vi "FP Server.vi"(8 "error in":errorcluster, 11 "FP Management In":refnum<class "Front Panel Manager.lvclass">) -> (0 "error out":errorcluster, 3 "FP Management Out":refnum<class "Front Panel Manager.lvclass">)   [LabVIEW 2015, in "Front Panel Publisher.lvlib" / "Front Panel Manager.lvclass"]
uses:
  Front Panel Manager.lvclass
  Websocket_class/Websocket.lvclass
  <vilib>/wsapi/NI_WebServices.lvlib
  Connection ID Methods.ctl
  FP Server Message.ctl
  Web Front Panel_class/Web Front Panel.lvclass
  <userlib>/_OpenG.lib/array/array.llb/Conditional Auto-Indexing Tunnel (String)__ogtk.vi
  <userlib>/_OpenG.lib/array/array.llb/Conditional Auto-Indexing Tunnel (U64)__ogtk.vi
panel:
  out "Stop Loop":bool
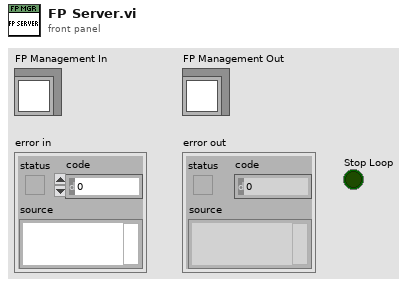
[diagram p1: front panel]
types:
  T1 = typedef "Front Panel Publisher.lvlib/Front Panel Manager.lvclass/Connection ID Methods.ctl" = enum16{"Read Data", "Write Connection ID", "Remove Connection ID"}
  T2 = typedef "Front Panel Publisher.lvlib/Front Panel Manager.lvclass/FP Server Message.ctl" = cluster{"Message":string, "Page":string, "Data":string[][], "Connection ID":u64, "Values and Position":refnum<vi>[]}
  T3 = typedef "FrontPanelPublisher.lvlib/FrontPanelManager.lvclass/FPServerMessage.ctl" = cluster{"Message":string, "Page":string, "Data":string[][], "Connection ID":u64, "Values and Position":refnum<vi>[]}
  T4 = typedef "Front Panel Publisher.lvlib/Web Front Panel.lvclass/High Level Config Settings.ctl" = cluster{"Default Refresh Rate (ms)":i32, "Show Border":bool, "Decorations Can Change":bool, "Synchronous Requests":bool, "Reduce Sent Data":bool}
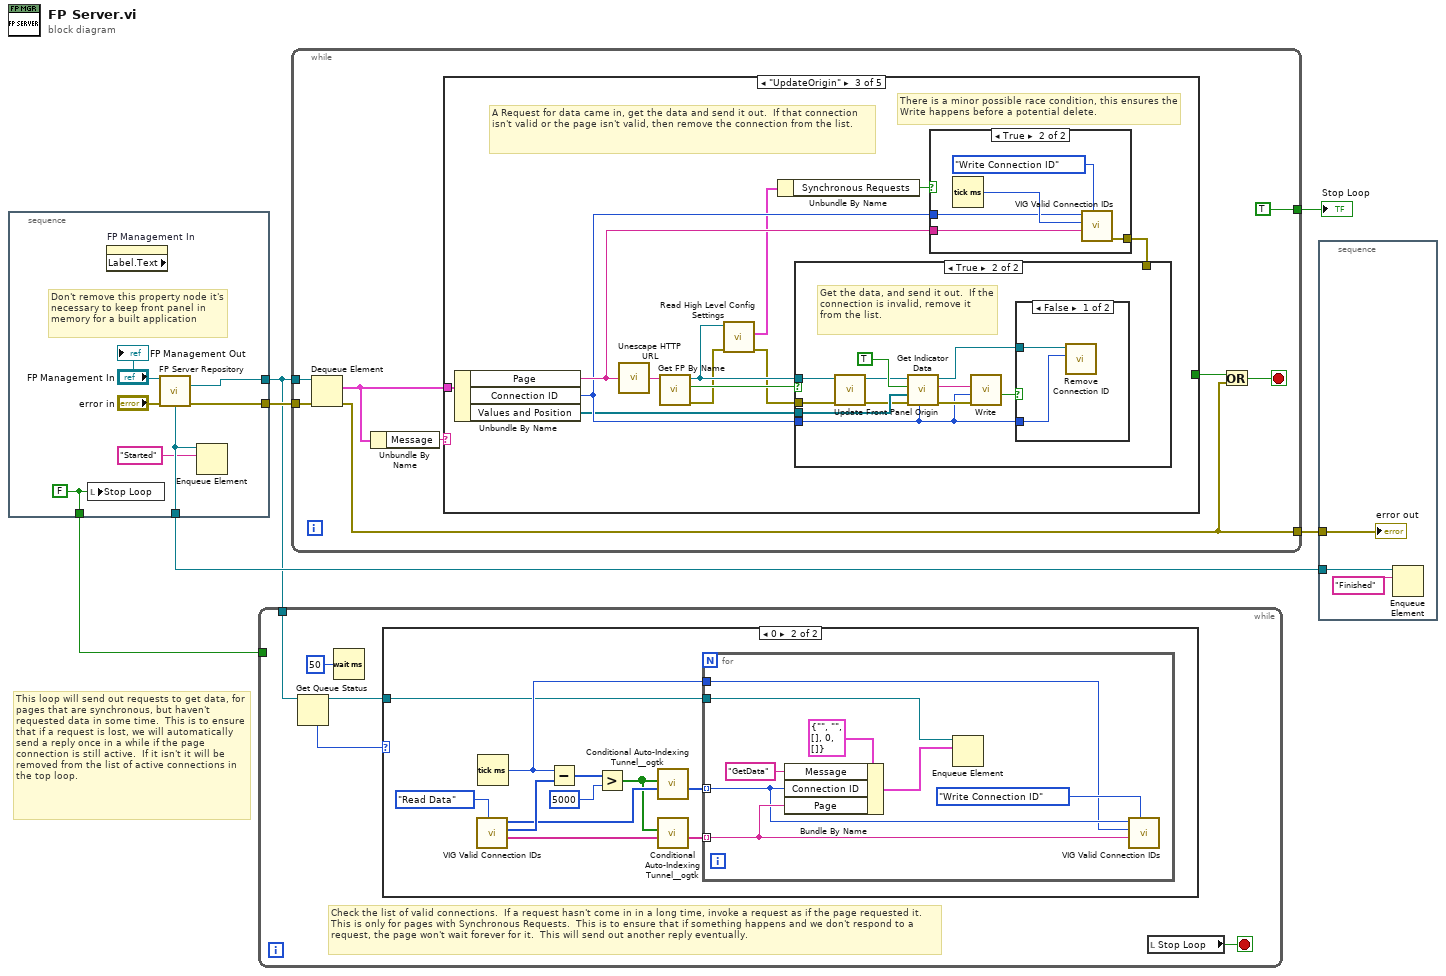
[diagram p0: block diagram]
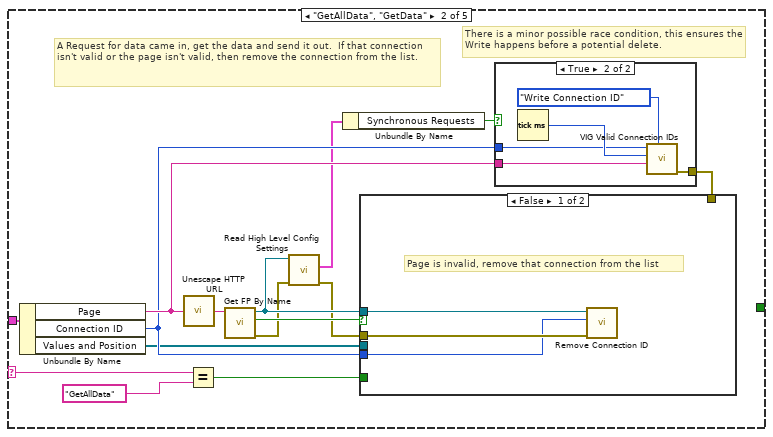
[diagram p3: hidden frame]
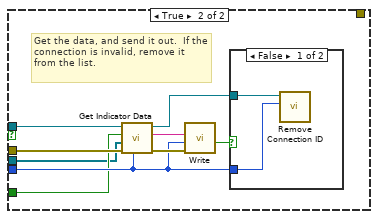
[diagram p5: hidden frame]
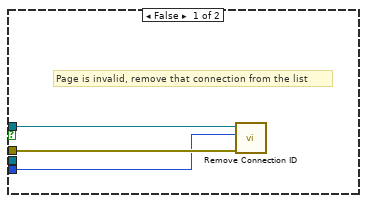
[diagram p8: hidden frame]
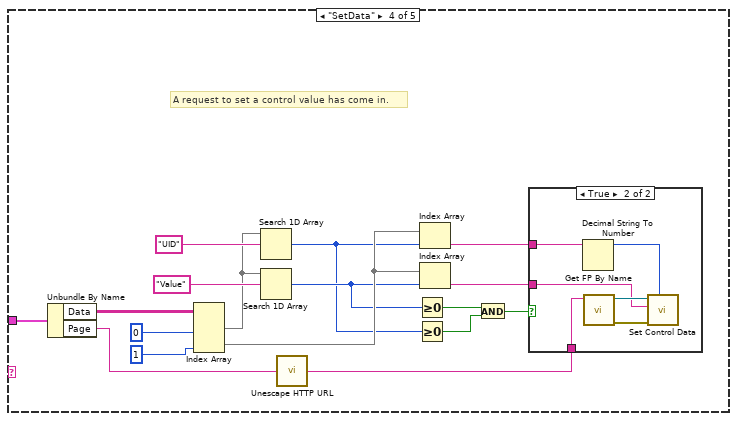
[diagram p10: hidden frame]
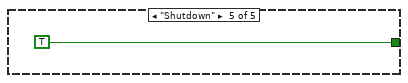
[diagram p12: hidden frame]
diagram:
  # "This loop will send out requests to get data, for pages that are synchronous, but haven't requested data in some time.  This is to ensure that if a request is lost, we will automatically send a reply once in a while if the page connection is still active.  If it isn't it will be removed from the list of active connections in the top loop."
  n1 = stacked-sequence {
    tunnel: [w11] -> w6
    tunnel: [w10] -> w3
    tunnel: [w8] -> w2
    tunnel: [w7] -> w4
    frame #0 {
      w7 = FALSE ("Stop Loop")
      # "Don't remove this property node it's necessary to keep front panel in memory for a built application"
      n2 = local write "Stop Loop"(w7) -> ()
      n3 = property on="FP Management In" class="LVClassControl (strict)" props=["Label", "Text"]() -> ()  [unwired: 2 in, 3 out]
      n4 = call "FP Server Repository.vi"("FP Management In"="FP Management In", "error in (no error)"="error in") -> ("ToProcessQueue"=w8:refnum<queue>, "ProcessSyncQueue"=w10:refnum<queue>, "error out"=w11:errorcluster)  [unwired: 7 in, 4 out]
      n5 = Enqueue Element(queue=w10, element="Started") -> ()  [unwired: 2 in, 3 out]
      "FP Management Out" <- "FP Management In"
    }
  }
  n6 = while {
    tunnel: w4 -> [_]
    tunnel: w2 -> [w16]
    stop <- w18 stop-if-true
    # "Check the list of valid connections.  If a request hasn't come in in a long time, invoke a request as if the page requested it.  This is only for pages with Synchronous Requests.  This is to ensure that if something happens and we don't respond to a request, the page won't wait forever for it.  This will send out another reply eventually."
    n7 = Get Queue Status(queue=w16) -> (queue out=w15:refnum<queue>, # elements in queue=w14:i32)  [unwired: 2 in, 6 out]
    n8 = Wait (ms)(milliseconds to wait=u32 50) -> ()  [unwired: 1 out]
    n9 = case shown="0" w14 {
      tunnel: w15 -> [_ w19]
      frame Default {
      }
      frame 0 {
        n10 = call "VIG Valid Connection IDs.vi"("Method (Read)"=Connection_ID_Methods."Read Data") -> ("Pages"=w22:string[], "Ticks"=w29:u32[], "Connections"=w26:u64[])  [unwired: 7 in, 1 out]
        n11 = Tick Count (ms)() -> (millisecond timer value=w20:u32)
        n12 = Subtract(x=w20, y=w29) -> (x-y=w28:u32[])
        n13 = Greater?(x=w28, y=u32 5000) -> (0:w23:bool[])
        n14 = call-poly <userlib>:"Conditional Auto-Indexing Tunnel__ogtk.vi"("Array in"=w26, "Elements to keep"=w23) -> ("Filtered Array out"=w25:u64[])  [unwired: 5 in]
        n15 = call-poly <userlib>:"Conditional Auto-Indexing Tunnel__ogtk.vi"("Array in"=w22, "Elements to keep"=w23) -> ("Filtered Array out"=w21:string[])  [unwired: 5 in]
        n16 = for {
          tunnel: w25 -> [w32] mode=indexing
          tunnel: w21 -> [w33] mode=indexing
          tunnel: w20 -> [w31]
          tunnel: w19 -> [w30]
          n17 = Bundle By Name(cluster=T2 {"Message"="", "Page"="", "Data"=[], "Connection ID"=0, "Values and Position"=[]} ("element"), "Message"="GetData", "Connection ID"=w32, "Page"=w33) -> (w35:T2)
          n18 = Enqueue Element(queue=w30, element=w35) -> ()  [unwired: 2 in, 3 out]
          n19 = call "VIG Valid Connection IDs.vi"("Method (Read)"=Connection_ID_Methods."Write Connection ID", "Page"=w33, "Tick Of Reply"=w31, "Connection ID"=w32) -> ()  [unwired: 4 in, 4 out]
        }
      }
    }
    n20 = local read "Stop Loop"() -> (w18:bool)
  }
  n21 = while {
    tunnel: w2 -> [w45]
    tunnel: [w39] -> w5
    tunnel: w6 -> [w42]
    tunnel: [TRUE] -> w1
    stop <- w40 stop-if-true
    n22 = Dequeue Element(queue=w45, error in (no error)=w42) -> (element=w41:T3, error out=w39:errorcluster)  [unwired: 1 in, 2 out]
    n23 = Unbundle By Name(w41) -> ("Message"=w44:string)
    n24 = case shown="\"UpdateOrigin\"" w44 {
      selector: w44 -> [_ w49 _ _ _]
      tunnel: [_ _ _ _ TRUE] -> w43
      tunnel: w41 -> [_ w60 w91 w114 _]
      frame Default {
      }
      frame "GetAllData", "GetData" {
        # "There is a minor possible race condition, this ensures the Write happens before a potential delete."
        # "A Request for data came in, get the data and send it out.  If that connection isn't valid or the page isn't valid, then remove the connection from the list."
        n25 = Unbundle By Name(w60) -> ("Page"=w54:string, "Connection ID"=w53:u64, "Values and Position"=w46:refnum<vi>[])
        n26 = call <vilib>:"Unescape HTTP URL.vi"("escaped string in"=w54) -> ("unescaped string out"=w58:string)
        n27 = Equal?(x=w49, y="GetAllData") -> (x = y?=w47:bool)
        n28 = call "Get FP By Name.vi"("WFP Name"=w58) -> ("error out"=w56:errorcluster, "Found"=w59:bool, "Web FP Out"=w57:refnum<class "Web Front Panel.lvclass">)  [unwired: 8 in]
        n29 = call "Read High Level Config Settings.vi"("error in (no error)"=w56, "Web FP In"=w57) -> ("error out"=w55:errorcluster, "High Level Config Settings"=w52:T4)  [unwired: 7 in, 1 out]
        n30 = Unbundle By Name(w52) -> ("Synchronous Requests"=w51:bool)
        n31 = case shown="True" w51 {
          tunnel: w54 -> [_ w63]
          tunnel: w53 -> [_ w62]
          tunnel: [_ w61] -> w50
          frame False {
          }
          frame True {
            n32 = Tick Count (ms)() -> (millisecond timer value=w64:u32)
            n33 = call "VIG Valid Connection IDs.vi"("Method (Read)"=Connection_ID_Methods."Write Connection ID", "Page"=w63, "Tick Of Reply"=w64, "Connection ID"=w62) -> ("error out"=w61:errorcluster)  [unwired: 4 in, 3 out]
          }
        }
        n34 = case shown="False" w59 {
          tunnel: w57 -> [w67 w77]
          tunnel: w55 -> [w68 w76]
          tunnel: w53 -> [w66 w72]
          tunnel: w50 -> [_ _]
          tunnel: w47 -> [_ w70]
          tunnel: w46 -> [_ w69]
          frame False {
            # "Page is invalid, remove that connection from the list"
            n35 = call "Remove Connection ID.vi"("error in (no error)"=w68, "Connection ID"=w66, "Web FP In"=w67) -> ()  [unwired: 8 in, 1 out]
          }
          frame True {
            # "Get the data, and send it out.  If the connection is invalid, remove it from the list."
            n36 = call-dynamic "Get Indicator Data.vi"("Connection ID"=w72, "error in (no error)"=w76, "Values and Position"=w69, "Get All"=w70, "Web FP In"=w77) -> ("error out"=w74:errorcluster, "String"=w75:string, "Web FP Out"=w71:refnum<class "Web Front Panel.lvclass">)  [unwired: 4 in]
            n37 = call "Write.vi"("error in (no error)"=w74, "Connection ID"=w72, "Payload"=w75) -> ("Connection Valid"=w73:bool)  [unwired: 6 in, 2 out]
            n38 = case shown="False" w73 {
              tunnel: w72 -> [w79 _]
              tunnel: w71 -> [w78 _]
              frame False {
                n39 = call "Remove Connection ID.vi"("Connection ID"=w79, "Web FP In"=w78) -> ()  [unwired: 9 in, 1 out]
              }
              frame True {
              }
            }
          }
        }
      }
      frame "UpdateOrigin" {
        # "There is a minor possible race condition, this ensures the Write happens before a potential delete."
        # "A Request for data came in, get the data and send it out.  If that connection isn't valid or the page isn't valid, then remove the connection from the list."
        n40 = Unbundle By Name(w91) -> ("Page"=w85:string, "Connection ID"=w84:u64, "Values and Position"=w80:refnum<vi>[])
        n41 = call <vilib>:"Unescape HTTP URL.vi"("escaped string in"=w85) -> ("unescaped string out"=w89:string)
        n42 = call "Get FP By Name.vi"("WFP Name"=w89) -> ("error out"=w87:errorcluster, "Found"=w90:bool, "Web FP Out"=w88:refnum<class "Web Front Panel.lvclass">)  [unwired: 8 in]
        n43 = call "Read High Level Config Settings.vi"("error in (no error)"=w87, "Web FP In"=w88) -> ("error out"=w86:errorcluster, "High Level Config Settings"=w83:T4)  [unwired: 7 in, 1 out]
        n44 = Unbundle By Name(w83) -> ("Synchronous Requests"=w82:bool)
        n45 = case shown="True" w82 {
          tunnel: w85 -> [_ w94]
          tunnel: w84 -> [_ w93]
          tunnel: [_ w92] -> w81
          frame False {
          }
          frame True {
            n46 = Tick Count (ms)() -> (millisecond timer value=w95:u32)
            n47 = call "VIG Valid Connection IDs.vi"("Method (Read)"=Connection_ID_Methods."Write Connection ID", "Page"=w94, "Tick Of Reply"=w95, "Connection ID"=w93) -> ("error out"=w92:errorcluster)  [unwired: 4 in, 3 out]
          }
        }
        n48 = case shown="True" w90 {
          tunnel: w88 -> [w98 w103]
          tunnel: w86 -> [w99 w100]
          tunnel: w84 -> [w97 w107]
          tunnel: w81 -> [_ _]
          tunnel: w80 -> [_ w105]
          frame False {
            # "Page is invalid, remove that connection from the list"
            n49 = call "Remove Connection ID.vi"("error in (no error)"=w99, "Connection ID"=w97, "Web FP In"=w98) -> ()  [unwired: 8 in, 1 out]
          }
          frame True {
            # "Get the data, and send it out.  If the connection is invalid, remove it from the list."
            n50 = call "Update Front Panel Origin.vi"("error in (no error)"=w100, "WebFrontPanel in"=w103) -> ("error out"=w102:errorcluster, "WebFrontPanel out"=w101:refnum<class "Web Front Panel.lvclass">)  [unwired: 8 in]
            n51 = call-dynamic "Get Indicator Data.vi"("Connection ID"=w107, "error in (no error)"=w102, "Values and Position"=w105, "Get All"=TRUE, "Web FP In"=w101) -> ("error out"=w109:errorcluster, "String"=w110:string, "Web FP Out"=w106:refnum<class "Web Front Panel.lvclass">)  [unwired: 4 in]
            n52 = call "Write.vi"("error in (no error)"=w109, "Connection ID"=w107, "Payload"=w110) -> ("Connection Valid"=w108:bool)  [unwired: 6 in, 2 out]
            n53 = case shown="False" w108 {
              tunnel: w107 -> [w112 _]
              tunnel: w106 -> [w111 _]
              frame False {
                n54 = call "Remove Connection ID.vi"("Connection ID"=w112, "Web FP In"=w111) -> ()  [unwired: 9 in, 1 out]
              }
              frame True {
              }
            }
          }
        }
      }
      frame "SetData" {
        # "A request to set a control value has come in."
        n55 = Unbundle By Name(w114) -> ("Data"=w115:string[][], "Page"=w116:string)
        n56 = Index Array(array=w115, index (col) #1=0 ("disabled index (col)"), index (col) #2=1 ("index (col)")) -> (element #1=w127:string[], element #2=w126:string[])  [unwired: 2 in]
        n57 = Search 1D Array(1D array=w127, element="UID") -> (index of element=w122:i32)  [unwired: 1 in]
        n58 = Search 1D Array(1D array=w127, element="Value") -> (index of element=w123:i32)  [unwired: 1 in]
        n59 = call <vilib>:"Unescape HTTP URL.vi"("escaped string in"=w116) -> ("unescaped string out"=w113:string)
        n60 = Greater Or Equal To 0?(x=w123) -> (x >= 0?=w121:bool)
        n61 = Greater Or Equal To 0?(x=w122) -> (x >= 0?=w120:bool)
        n62 = Index Array(array=w126, index=w122) -> (element=w125:string)
        n63 = Index Array(array=w126, index=w123) -> (element=w124:string)
        n64 = And(x=w121, y=w120) -> (x .and. y?=w119:bool)
        n65 = case shown="True" w119 {
          tunnel: w125 -> [_ w132]
          tunnel: w124 -> [_ w131]
          tunnel: w113 -> [_ w130]
          frame False {
          }
          frame True {
            n66 = Decimal String To Number(string=w132) -> (number=w134:i32)  [unwired: 2 in, 1 out]
            n67 = call "Get FP By Name.vi"("WFP Name"=w130) -> ("error out"=w133:errorcluster, "Web FP Out"=w135:refnum<class "Web Front Panel.lvclass">)  [unwired: 8 in, 1 out]
            n68 = call-dynamic "Set Control Data.vi"("UID"=w134, "error in (no error)"=w133, "Value"=w131, "Web FP In"=w135) -> ()  [unwired: 6 in, 2 out]
          }
        }
      }
      frame "Shutdown" {
      }
    }
    n69 = Or(x=w43, y=w39) -> (x .or. y?=w40:bool)
  }
  "Stop Loop" <- w1
  n70 = stacked-sequence {
    tunnel: w5 -> [w139]
    tunnel: w3 -> [w138]
    frame #0 {
      n71 = Enqueue Element(queue=w138, element="Finished") -> ()  [unwired: 2 in, 3 out]
      "error out" <- w139
    }
  }
